vi "parseResponse.vi"(8 "error in (no error)":errorcluster, 10 "response in":string, 11 "CoolerSerialCommand in":refnum<class "CoolerSerialCommand.lvclass">) -> (0 "error out":errorcluster, 2 "response out":T1, 3 "CoolerSerialCommand out":refnum<class "CoolerSerialCommand.lvclass">)   [LabVIEW 2016, in "CoolerSerialCommand.lvclass"]
uses:
  CoolerSerialCommand.lvclass
  typedefs/response.ctl
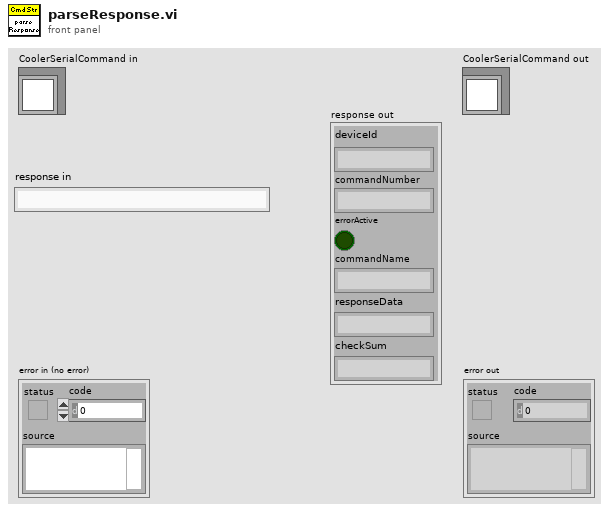
[diagram p1: front panel]
types:
  T1 = typedef "response.ctl" = cluster{"deviceId":string, "commandNumber":string, "errorActive":bool, "commandName":string, "responseData":string, "checkSum":string}
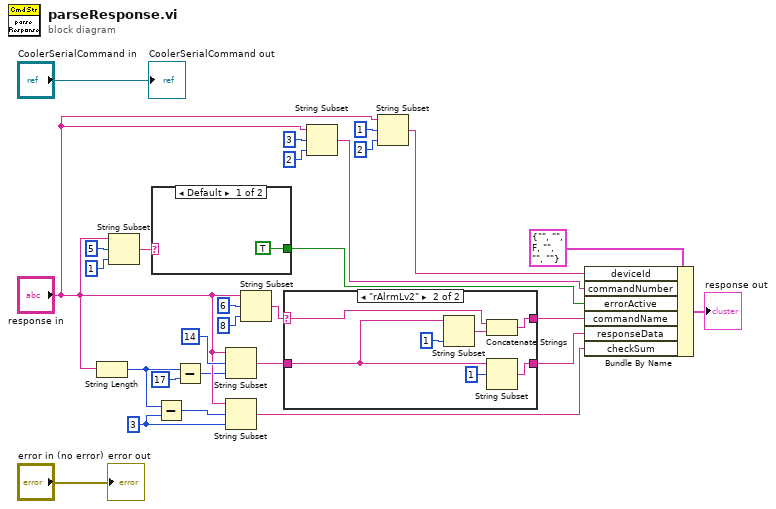
[diagram p0: block diagram]
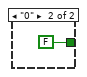
[diagram p3: hidden frame]
diagram:
  w6 = 3 ("offset (0)")
  n1 = String Length(string="response in") -> (length=w7:i32)
  n2 = String Subset(string="response in", offset (0)=5, length (rest)=1 ("offset (0)")) -> (substring=w13:string)
  n3 = case shown="Default" w13 {
    tunnel: [TRUE ("errorActive") FALSE ("errorActive")] -> w12
    frame Default {
    }
    frame "0" {
    }
  }
  n4 = Subtract(x=w7, y=w6) -> (x-y=w8:i32)
  n5 = Subtract(x=w7, y=17) -> (x-y=w9:i32)
  n6 = String Subset(string="response in", offset (0)=14, length (rest)=w9) -> (substring=w5:string)
  n7 = String Subset(string="response in", offset (0)=w8, length (rest)=w6) -> (substring=w24:string)
  n8 = String Subset(string="response in", offset (0)=6, length (rest)=8 ("offset (0)")) -> (substring=w3:string)
  n9 = case shown="\"rAlrmLv2\"" w3 {
    selector: w3 -> [w32 w35]
    tunnel: [w31 w38] -> w1
    tunnel: w5 -> [w31 w33]
    tunnel: [w32 w39] -> w2
    frame Default {
    }
    frame "rAlrmLv2" {
      n10 = String Subset(string=w33, length (rest)=1 ("length (rest)")) -> (substring=w36:string)  [unwired: 1 in]
      n11 = Concatenate Strings(w35, w36) -> (w39:string)
      n12 = String Subset(string=w33, offset (0)=1) -> (substring=w38:string)  [unwired: 1 in]
    }
  }
  n13 = String Subset(string="response in", offset (0)=3, length (rest)=2 ("offset (0)")) -> (substring=w4:string)
  n14 = String Subset(string="response in", offset (0)=1, length (rest)=2 ("offset (0)")) -> (substring=w23:string)
  n15 = Bundle By Name(cluster=T1 {"deviceId"="", "commandNumber"="", "errorActive"=FALSE, "commandName"="", "responseData"="", "checkSum"=""} ("response out"), "deviceId"=w23, "commandNumber"=w4, "errorActive"=w12, "commandName"=w2, "responseData"=w1, "checkSum"=w24) -> (→"response out":T1)
  "error out" <- "error in (no error)"
  "CoolerSerialCommand out" <- "CoolerSerialCommand in"
